vi "update_disk_spinning.vi"(2 "error in (no error)":errorcluster, 4 "disk spinning":bool, 5 "VISA resource name":refnum<visa-resource-name>) -> (0 "error out":errorcluster, 1 "VISA resource name out":refnum<visa-resource-name>)   [LabVIEW 2016]
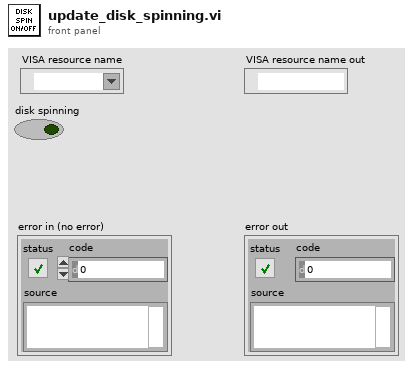
[diagram p1: front panel]
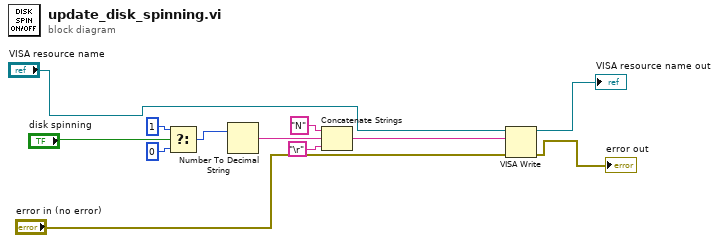
[diagram p0: block diagram]
diagram:
  n1 = Select(t=i8 1, s="disk spinning", f=i8 0) -> (s? t:f=w5:i8)
  n2 = Number To Decimal String(number=w5) -> (decimal integer string=w12:string)  [unwired: 1 in]
  n3 = Concatenate Strings("N" ("string"), w12, "\r") -> (w9:string)
  n4 = VISA Write(VISA resource name="VISA resource name", write buffer=w9, error in (no error)="error in (no error)") -> (VISA resource name out=→"VISA resource name out":refnum<visa-resource-name>, error out=→"error out":errorcluster)  [unwired: 1 out]
